vi "ControlReference.FGV.vi"(7 "pathToMainVI":path, 8 "error in (no error)":errorcluster, 10 "state (getReference)":T1=enum."getReference", 11 "controlLabelText":string) -> (0 "error out":errorcluster, 1 "referenceToControl":refnum<vi>)   [LabVIEW 2019]
uses:
  State.ctl
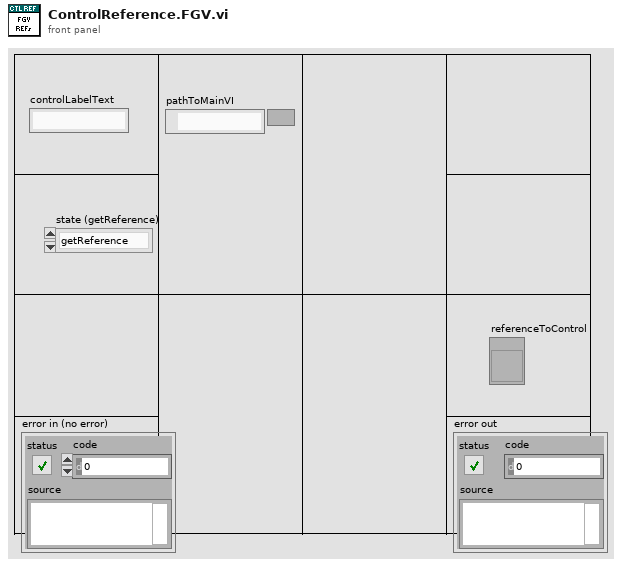
[diagram p1: front panel]
types:
  T1 = typedef "State.ctl" = enum16{"setReferences", "getReference", "closeReferences"}
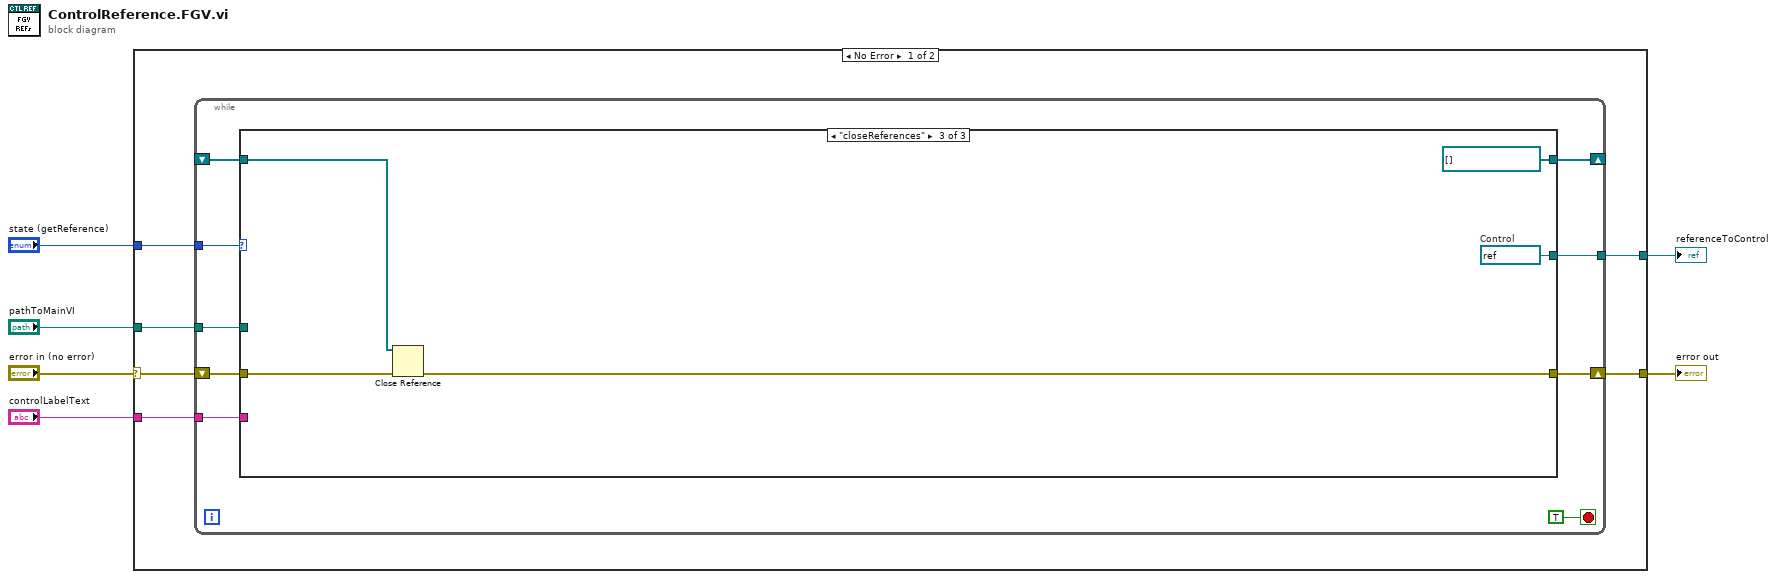
[diagram p0: block diagram]
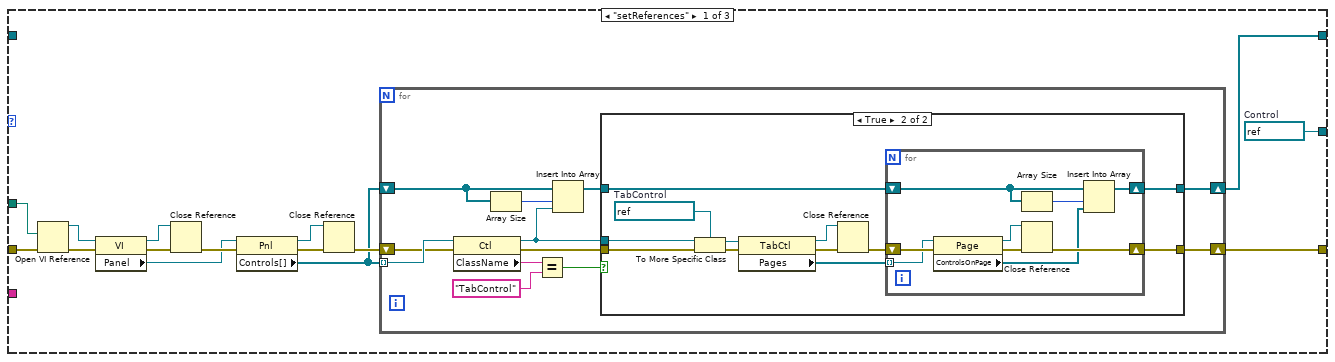
[diagram p2: hidden frame]
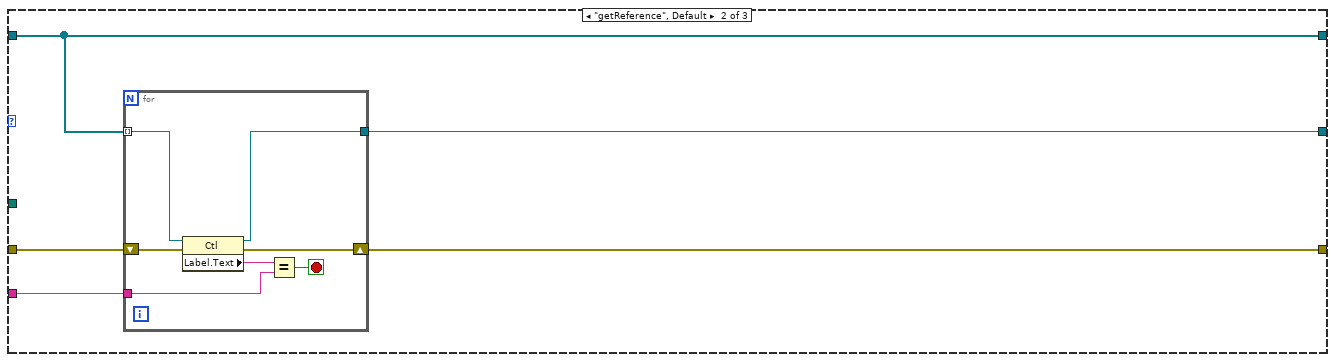
[diagram p4: hidden frame]
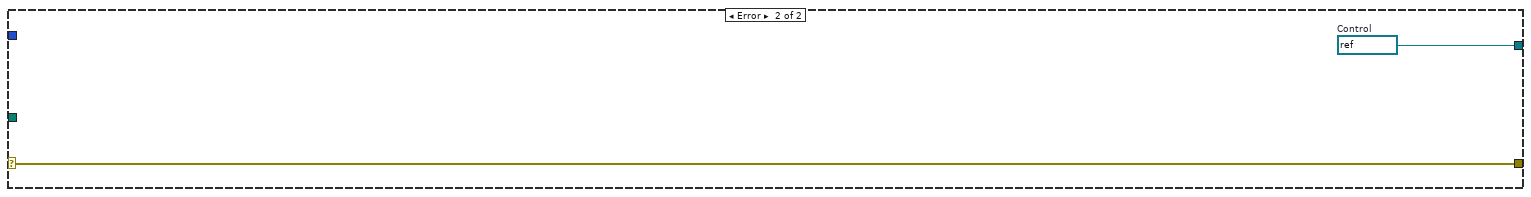
[diagram p5: hidden frame]
diagram:
  n1 = case shown="No Error" "error in (no error)" {
    selector: "error in (no error)" -> [w10 w90]
    tunnel: [w12 w90] -> w6
    tunnel: "pathToMainVI" -> [w11 _]
    tunnel: "state (getReference)" -> [w9 _]
    tunnel: "controlLabelText" -> [w8 _]
    tunnel: [w7 w89] -> w1
    frame No Error {
      n2 = while {
        tunnel: w11 -> [w20]
        shift-right: [w21] -> w12
        shift-left: w10 -> [w18]
        tunnel: w9 -> [w17]
        shift-right: [w15] -> _
        shift-left: _ -> [w16]
        tunnel: w8 -> [w14]
        tunnel: [w13] -> w7
        stop <- TRUE stop-if-true
        n3 = case shown="\"closeReferences\"" w17 {
          tunnel: [w29 w74 w87] -> w21
          tunnel: w20 -> [w28 _ _]
          tunnel: w18 -> [w25 w76 w88]
          tunnel: w16 -> [_ w75 w86]
          tunnel: [w23 w75 refnum<vi>[] [] ("Controls[]")] -> w15
          tunnel: w14 -> [_ w73 _]
          tunnel: [w22 w72 w84] -> w13
          frame "setReferences" {
            w22 = refnum<vi> refnum  # Control
            n4 = Open VI Reference(vi path=w28, error in (no error)=w25) -> (vi reference=w26:refnum<vi>, error out=w27:errorcluster)  [unwired: 4 in]
            n5 = property class="VI"(reference=w26, error in=w27) -> (reference out=w35:refnum<vi>, error out=w36:errorcluster, "Panel"=w33:refnum<vi>)
            n6 = Close Reference(reference=w35, error in (no error)=w36) -> (error out=w34:errorcluster)
            n7 = property class="Pnl"(reference=w33, error in=w34) -> (reference out=w32:refnum<vi>, error out=w31:errorcluster, "Controls[]"=w24:refnum<vi>[])
            n8 = Close Reference(reference=w32, error in (no error)=w31) -> (error out=w30:errorcluster)
            n9 = for {
              shift-right: [w44] -> w29
              shift-left: w30 -> [w47]
              tunnel: w24 -> [w48] mode=indexing
              shift-right: [w42] -> w23
              shift-left: w24 -> [w41]
              n10 = property class="Ctl"(reference=w48, error in=w47) -> (reference out=w38:refnum<vi>, error out=w37:errorcluster, "ClassName"=w46:string)
              n11 = Array Size(array=w41) -> (size(s)=w39:i32)
              n12 = Equal?(x=w46, y="TabControl") -> (x = y?=w43:bool)
              n13 = Insert Into Array(array=w41, index=w39, new element=w38) -> (w40:refnum<vi>[])
              n14 = case shown="True" w43 {
                tunnel: [w50 w54] -> w44
                tunnel: w37 -> [w50 w61]
                tunnel: w38 -> [_ w62]
                tunnel: [w49 w52] -> w42
                tunnel: w40 -> [w49 w51]
                frame False {
                }
                frame True {
                  w59 = refnum<vi> refnum  # TabControl
                  n15 = To More Specific Class(target class=w59, reference=w62, error in=w61) -> (specific class reference=w58:refnum<vi>, error out=w60:errorcluster)
                  n16 = property class="TabCtl"(reference=w58, error in=w60) -> (reference out=w57:refnum<vi>, error out=w56:errorcluster, "Pages"=w53:refnum<vi>[])
                  n17 = Close Reference(reference=w57, error in (no error)=w56) -> (error out=w55:errorcluster)
                  n18 = for {
                    shift-right: [w68] -> w54
                    shift-left: w55 -> [w71]
                    tunnel: w53 -> [w70] mode=indexing
                    shift-right: [w65] -> w52
                    shift-left: w51 -> [w63]
                    n19 = property class="Page"(reference=w70, error in=w71) -> (reference out=w67:refnum<vi>, error out=w69:errorcluster, "ControlsOnPage"=w66:refnum<vi>[])
                    n20 = Array Size(array=w63) -> (size(s)=w64:i32)
                    n21 = Close Reference(reference=w67, error in (no error)=w69) -> (error out=w68:errorcluster)
                    n22 = Insert Into Array(array=w63, index=w64, new element=w66) -> (w65:refnum<vi>[])
                  }
                }
              }
            }
          }
          frame "getReference", Default {
            n23 = for {
              shift-right: [w81] -> w74
              shift-left: w76 -> [w83]
              tunnel: w75 -> [w82] mode=indexing
              tunnel: w73 -> [w79]
              tunnel: [w77] -> w72
              stop <- w78 stop-if-true
              n24 = property class="Ctl"(reference=w82, error in=w83) -> (reference out=w77:refnum<vi>, error out=w81:errorcluster, "Label.Text"=w80:string)
              n25 = Equal?(x=w80, y=w79) -> (x = y?=w78:bool)
            }
          }
          frame "closeReferences" {
            w84 = refnum<vi> refnum  # Control
            n26 = Close Reference(reference=w86, error in (no error)=w88) -> (error out=w87:errorcluster)
          }
        }
      }
    }
    frame Error {
      w89 = refnum<vi> refnum  # Control
    }
  }
  "error out" <- w6
  "referenceToControl" <- w1
